vi "Histogram2D2002.vi"   [LabVIEW 2013]
uses:
  <vilib>/Heliosphere Research LLC/Advanced Plotting Toolkit/api_plotting/Histogram2D_Automatic.vi
  <vilib>/Heliosphere Research LLC/Advanced Plotting Toolkit/Advanced Plotting Toolkit.lvlib
types:
  T1 = typedef "Advanced Plotting Toolkit.lvlib/PlotID.ctl" = i32
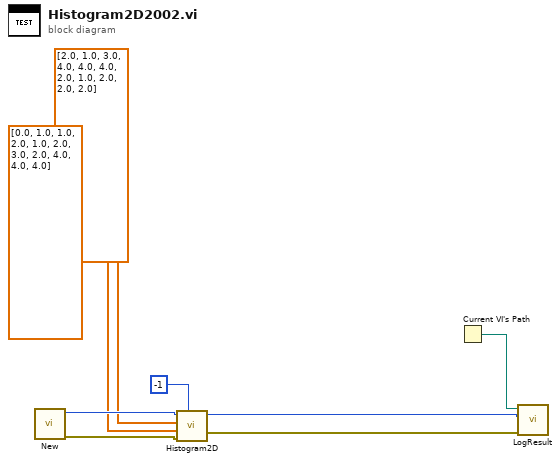
[diagram p0: block diagram]
diagram:
  n1 = call <vilib>:"New.vi"() -> ("error out"=w6:errorcluster, "Plot ID"=w7:T1)  [unwired: 10 in]
  n2 = call-poly <vilib>:"Histogram2D.vi"("X Bins"=-1, "error in (no error)"=w6, "Y Data"=dbl[] [2.0, 1.0, 3.0, 4.0, 4.0, 4.0, 2.0, 1.0, 2.0, 2.0, 2.0] ("X Data"), "X Data"=dbl[] [0.0, 1.0, 1.0, 2.0, 1.0, 2.0, 3.0, 2.0, 4.0, 4.0, 4.0], "Plot ID"=w7) -> ("error out"=w4:errorcluster, "Plot ID Out"=w5:T1)  [unwired: 5 in]
  n3 = Current VI's Path() -> (path=w8:path)
  n4 = call "LogResult.vi"("Test Result"=w4, "Test Artifact"=w5, "VI Path"=w8) -> ()  [unwired: 9 in]
